vi "Polynomial.vi"(0 "A":dbl, 1 "BX":dbl, 2 "CX^2":dbl, 3 "DX^3":dbl, 4 "EX^4":dbl, 5 "FX^5":dbl, 6 "X":dbl) -> (16 "Y":dbl)   [LabVIEW 2015]
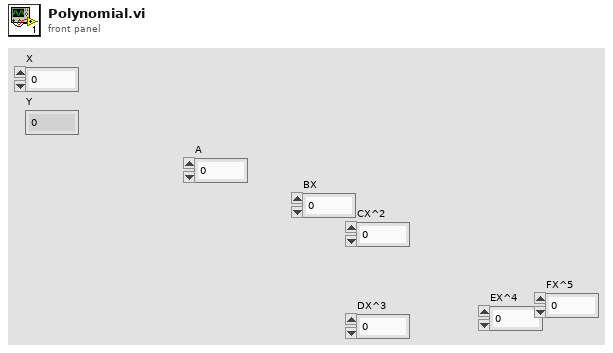
[diagram p1: front panel]
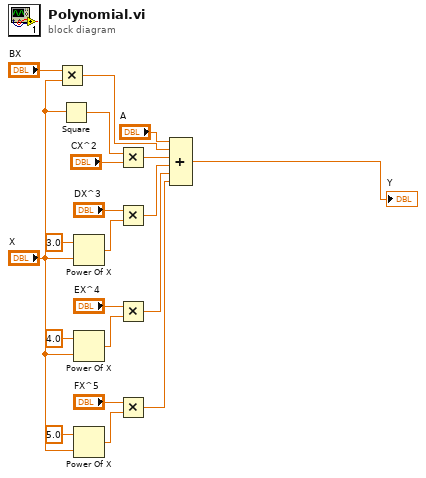
[diagram p0: block diagram]
diagram:
  n1 = Multiply(x="BX", y="X") -> (x*y=w18:dbl)
  n2 = Square(x="X") -> (x^2=w17:dbl)
  n3 = Power Of X(1:"X", 2:3.0 ("y")) -> (0:w14:dbl)
  n4 = Power Of X(1:"X", 2:4.0 ("y")) -> (0:w11:dbl)
  n5 = Power Of X(1:"X", 2:5.0 ("y")) -> (0:w8:dbl)
  n6 = Multiply(x=w17, y="CX^2") -> (x*y=w5:dbl)
  n7 = Multiply(x="DX^3", y=w14) -> (x*y=w4:dbl)
  n8 = Multiply(x="EX^4", y=w11) -> (x*y=w3:dbl)
  n9 = Multiply(x="FX^5", y=w8) -> (x*y=w2:dbl)
  n10 = Compound Arithmetic op=ADD("A", w18, w5, w4, w3, w2) -> (→"Y":dbl)
